vi "Logging Main.vi"() -> ()   [LabVIEW 2013]
doc: "This Continuous Measurement sample project is based on the Queued Message Handler template.\n\nThe Event Handling Loop generates messages based on user interface actions.\n\nThe Message Handling Loop processes messages generated by the Event Handling Loop, or by other messages. There are also Acquisition and Logging message handling loop subVIs, and a chart updating loop."
uses:
  Settings/Settings.ctl
  Acquisition/Hardware Configuration.ctl
  Acquisition/Signal Type.ctl
  Logging/Logging Configuration.ctl
  controls/Logging UI Data.ctl
  controls/Logging UI State.ctl
  support/Message Queue/Enqueue Message (Single).vi
  support/Message Queue/Enqueue Message (Array).vi
  <vilib>/Utility/error.llb/Error Cluster From Error Code.vi
  <vilib>/ErrorRing/Error Ring.xnode
  Acquisition/Logging Acquisition.lvlib
  Logging/Logging Logging.lvlib
  Settings/Logging Settings.lvlib
  support/User Event - Stop/Logging User Event - Stop.lvlib
  support/Message Queue/Logging Message Queue.lvlib
panel:
  out "Data":waveform(dbl)[](graph)
  in  "Settings":bool
  in  "Start":bool
  in  "Stop":bool
  out "Status":string
  in  "Exit":bool
  # "Continuous Measurement Data Logger"
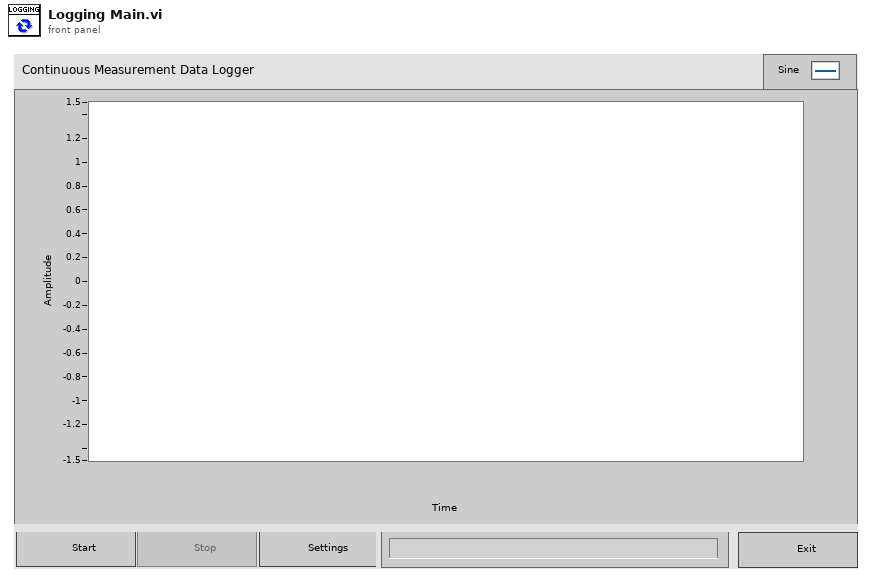
[diagram p1: front panel]
types:
  T1 = typedef "Logging UI State.ctl" = enum16{"Idle", "Acquiring and Logging", "Waiting for Exit", "Waiting for Exit (Acq Stopped)", "Waiting for Exit (Log Stopped)", "Waiting for Stop", "Waiting for Stop (Acq Stopped)", "Waiting for Stop (Log Stopped)"}
  T2 = typedef "Logging UI Data.ctl" = cluster{"Start Ref":refnum<vi>, "Stop Ref":refnum<vi>, "Settings Ref":refnum<vi>, "Exit Ref":refnum<vi>, "Status Ref":refnum<vi>, "Data Ref":refnum<vi>}
  T3 = typedef "Logging Settings.lvlib/Settings.ctl" = cluster{"Hardware Configuration":T4, "Logging Configuration":T6}
  T4 = typedef "Logging Acquisition.lvlib/Hardware Configuration.ctl" = cluster{"HW Refnum <Replace Me>":string, "Signal Type <Replace Me>":T5}
  T5 = typedef "Logging Acquisition.lvlib/Signal Type.ctl" = enum16{"Sine Wave", "Square with Noise"}
  T6 = typedef "Logging Logging.lvlib/Logging Configuration.ctl" = cluster{"Log File Base Path":path, "TDMS File Reference":refnum<k34>}
  T7 = typedef "Logging Message Queue.lvlib/All Message Queues.ctl" = cluster{"UI":refnum<queue>, "Acquisition":refnum<queue>, "Logging":refnum<queue>}
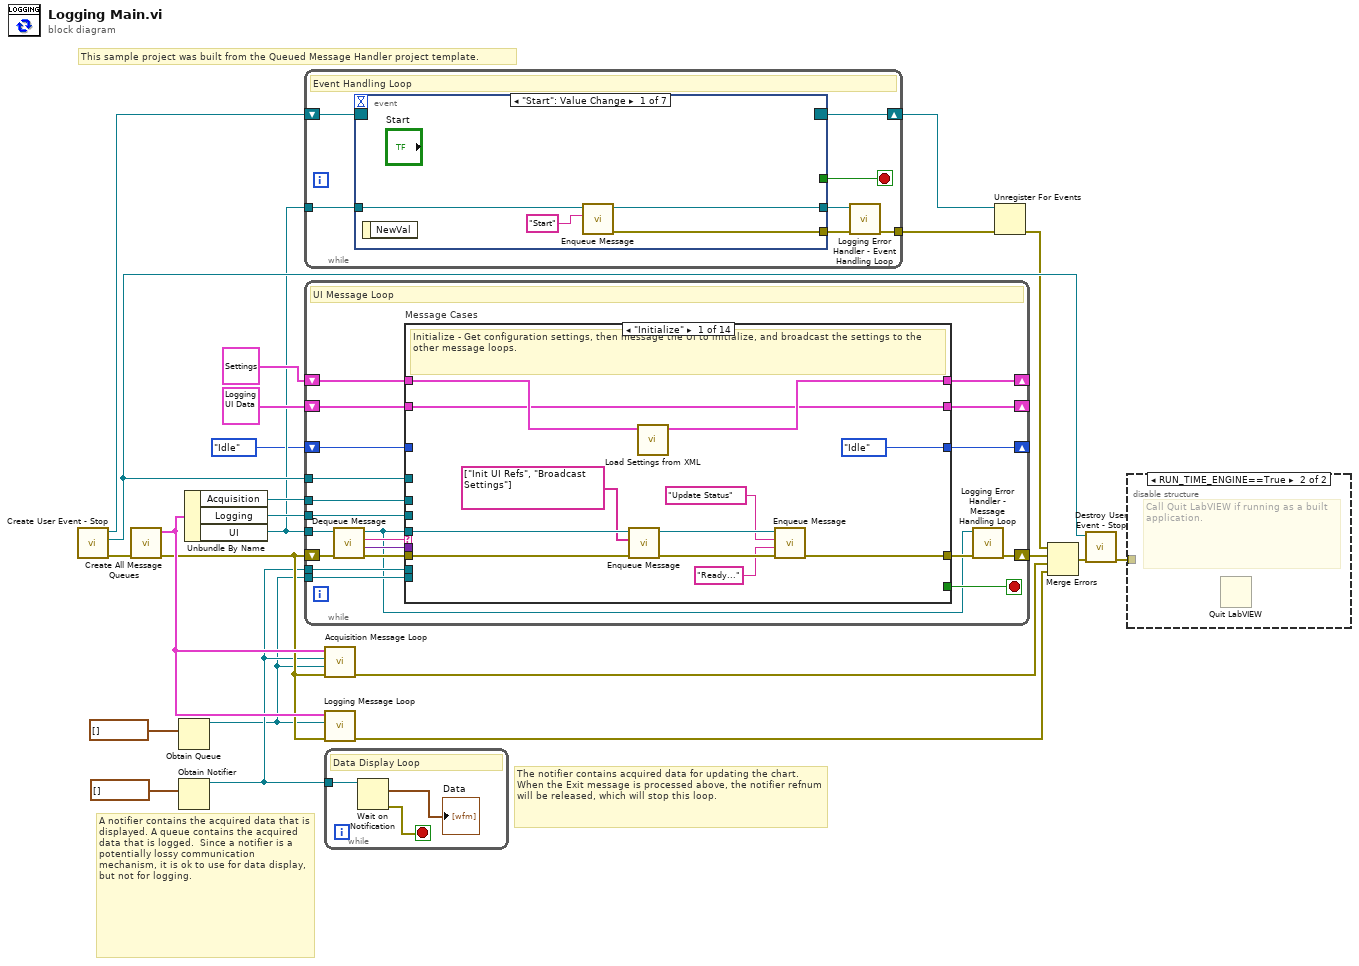
[diagram p0: block diagram]
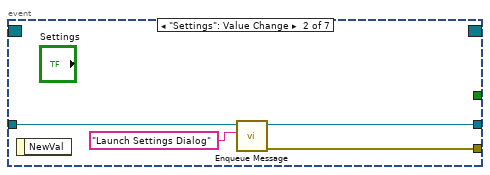
[diagram p3: hidden frame]
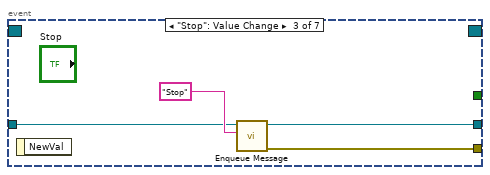
[diagram p4: hidden frame]
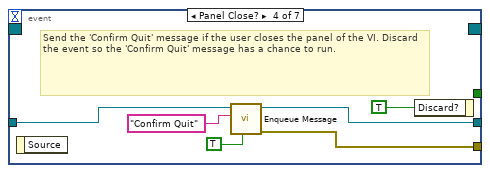
[diagram p5: hidden frame]
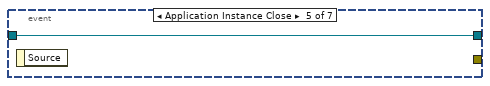
[diagram p6: hidden frame]
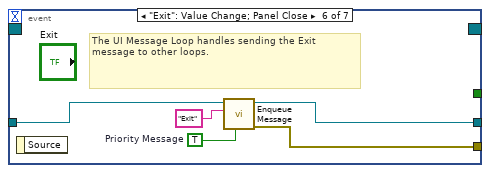
[diagram p7: hidden frame]
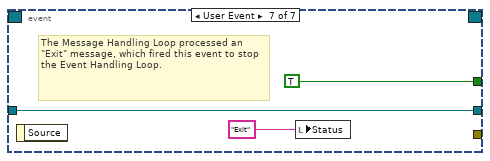
[diagram p8: hidden frame]
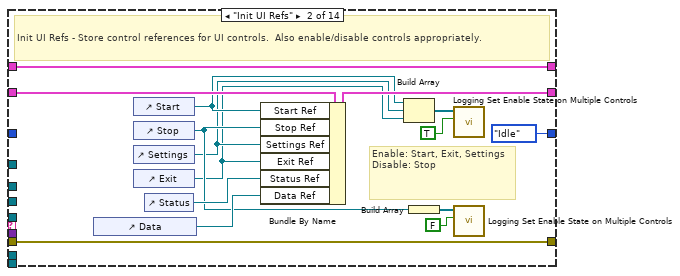
[diagram p9: hidden frame]
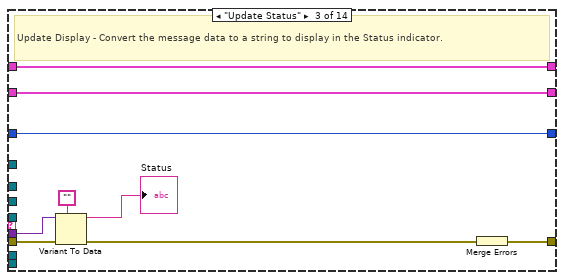
[diagram p10: hidden frame]
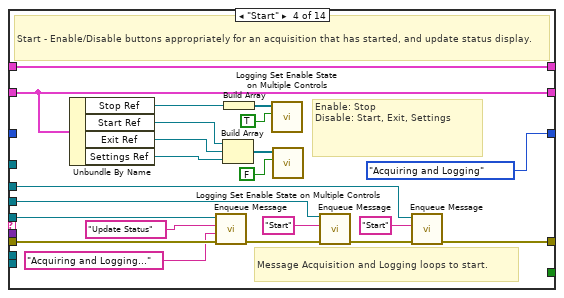
[diagram p11: hidden frame]
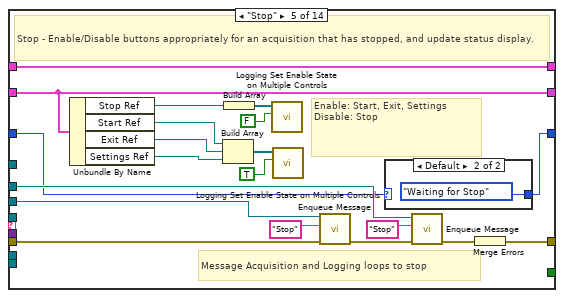
[diagram p12: hidden frame]
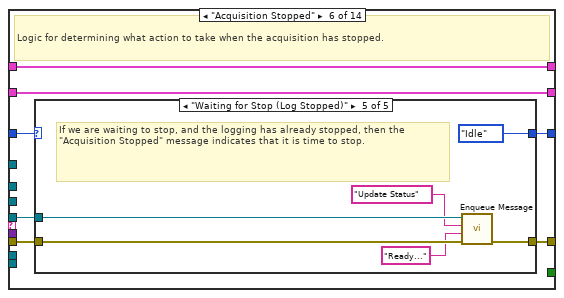
[diagram p14: hidden frame]
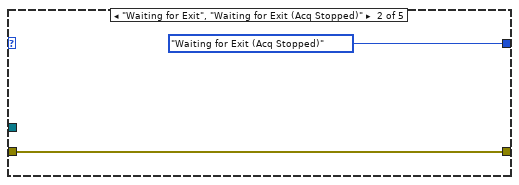
[diagram p16: hidden frame]
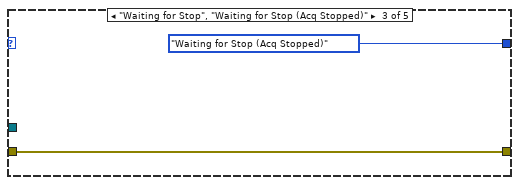
[diagram p17: hidden frame]
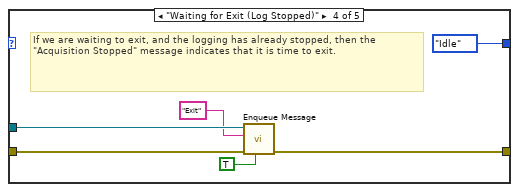
[diagram p18: hidden frame]
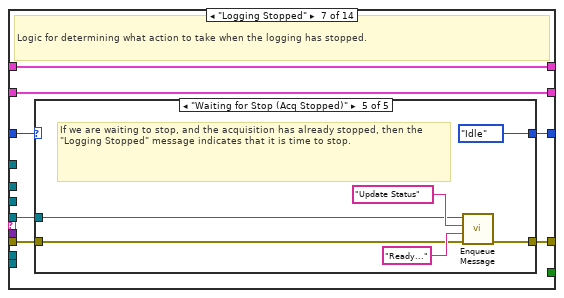
[diagram p19: hidden frame]
diagram:
  # "This sample project was built from the Queued Message Handler project template."
  # "A notifier contains the acquired data that is displayed. A queue contains the acquired data that is logged.  Since a notifier is a potentially lossy communication mechanism, it is ok to use for data display, but not for logging."
  # "The notifier contains acquired data for updating the chart. When the Exit message is processed above, the notifier refnum will be released, which will stop this loop."
  n1 = call "Create User Event - Stop.vi"() -> ("error out"=w18:errorcluster, "User Event - Stop"=w20:refnum<user-event>, "Stop Event Registration Refnum"=w21:refnum<event-registration>)  [unwired: 9 in]
  n2 = call "Create All Message Queues.vi"("error in (no error)"=w18) -> ("error out"=w15:errorcluster, "Message Queues out"=w17:T7)  [unwired: 9 in]
  n3 = Obtain Queue(element data type=waveform(dbl)[] []) -> (queue out=w4:refnum<queue>)  [unwired: 4 in, 2 out]
  n4 = Obtain Notifier(notification data type=waveform(dbl)[] []) -> (notifier out=w6:refnum<notifier>)  [unwired: 3 in, 2 out]
  n5 = Unbundle By Name(w17) -> ("Acquisition"=w10:refnum<queue>, "Logging"=w9:refnum<queue>, "UI"=w8:refnum<queue>)
  n6 = while {
    tunnel: w8 -> [w29]
    tunnel: [w26] -> w22
    shift-right: [w28] -> w12
    shift-left: w21 -> [w30]
    stop <- w27 stop-if-true
    # "Event Handling Loop"
    n7 = event shown="[0] \"Start\": Value Change" {
      selector: w30 -> [_ _ _ _ _ _ _]
      dyn-events: [_ _ _ _ _ _ _] -> w28
      timeout: _ -> [_ _ _ _ _ _ _]
      tunnel: [_ _ _ _ _ _ TRUE ("Discard?")] -> w27
      tunnel: w29 -> [w34 w36 w41 w46 w49 w51 w55]
      tunnel: [w32 w38 w40 w44 _ w54 _] -> w25
      tunnel: [w31 w35 w39 w45 w49 w50 w55] -> w24
      event "Start": Value Change {
        n8 = event-data() -> ()  [unwired: 1 in, 1 out]
        n9 = call-poly "Enqueue Message.vi"("Message"="Start", "Message Queue"=w34) -> ("error out"=w32:errorcluster, "dup Message Queue"=w31:refnum<queue>)  [unwired: 8 in]
      }
      event "Settings": Value Change {
        n10 = event-data() -> ()  [unwired: 1 in, 1 out]
        n11 = call-poly "Enqueue Message.vi"("Message"="Launch Settings Dialog", "Message Queue"=w36) -> ("error out"=w38:errorcluster, "dup Message Queue"=w35:refnum<queue>)  [unwired: 8 in]
      }
      event "Stop": Value Change {
        n12 = event-data() -> ()  [unwired: 1 in, 1 out]
        n13 = call-poly "Enqueue Message.vi"("Message"="Stop", "Message Queue"=w41) -> ("error out"=w40:errorcluster, "dup Message Queue"=w39:refnum<queue>)  [unwired: 8 in]
      }
      event Panel Close? {
        # "Send the 'Confirm Quit' message if the user closes the panel of the VI. Discard the event so the 'Confirm Quit' message has a chance to run."
        n14 = event-data() -> ()  [unwired: 1 in, 1 out]
        n15 = call-poly "Enqueue Message.vi"("Priority Message? (F)"=TRUE, "Message"="Confirm Quit", "Message Queue"=w46) -> ("error out"=w44:errorcluster, "dup Message Queue"=w45:refnum<queue>)  [unwired: 7 in]
        n16 = event-data("Discard?"=TRUE) -> ()  [unwired: 1 in, 1 out]
      }
      event Application Instance Close {
        n17 = event-data() -> ()  [unwired: 1 in, 1 out]
      }
      event "Exit": Value Change; Panel Close {
        w52 = TRUE  # Priority Message
        # "The UI Message Loop handles sending the Exit message to other loops."
        n18 = event-data() -> ()  [unwired: 1 in, 1 out]
        n19 = call-poly "Enqueue Message.vi"("Priority Message? (F)"=w52, "Message"="Exit", "Message Queue"=w51) -> ("error out"=w54:errorcluster, "dup Message Queue"=w50:refnum<queue>)  [unwired: 7 in]
      }
      event User Event {
        # "The Message Handling Loop processed an \"Exit\" message, which fired this event to stop the Event Handling Loop."
        n20 = event-data() -> ()  [unwired: 1 in, 1 out]
        n21 = local write "Status"("Exit" ("Exit String")) -> ()
      }
    }
    n22 = call "Logging Error Handler - Event Handling Loop.vi"("error in (no error)"=w25, "Message Queue"=w24) -> ("dup error in"=w26:errorcluster)  [unwired: 8 in, 1 out]
  }
  n23 = while {
    tunnel: w8 -> [w71]
    tunnel: w20 -> [w76]
    shift-right: [w62] -> w23
    shift-left: w15 -> [w75]
    shift-right: [w70] -> _
    shift-left: T3 {"Hardware Configuration"={"HW Refnum <Replace Me>"="", "Signal Type <Replace Me>"=enum."Sine Wave"}, "Logging Configuration"={"Log File Base Path"=path "", "TDMS File Reference"=refnum}} ("Settings") -> [w69]
    shift-right: [w67] -> _
    shift-left: T2 {"Start Ref"=refnum, "Stop Ref"=refnum, "Settings Ref"=refnum, "Exit Ref"=refnum, "Status Ref"=refnum, "Data Ref"=refnum} ("Measurement UI Controls") -> [w68]
    tunnel: w10 -> [w66]
    tunnel: w9 -> [w65]
    tunnel: w6 -> [w64]
    tunnel: w4 -> [w63]
    shift-right: [w58] -> _
    shift-left: Logging_UI_State."Idle" ("UI State") -> [w59]
    stop <- w77 stop-if-true
    # "UI Message Loop"
    n24 = call "Dequeue Message.vi"("error in (no error)"=w75, "Message Queue"=w71) -> ("error out"=w74:errorcluster, "Message Data"=w72:variant, "Message"=w73:string, "dup Message Queue"=w60:refnum<queue>)  [unwired: 6 in]
    n25 = case "Message Cases" shown="\"Initialize\"" w73 {
      selector: w73 -> [_ _ _ _ _ _ _ _ _ _ _ _ _ w298]
      tunnel: w60 -> [w81 _ _ w135 _ w160 w185 _ w225 w239 w250 w281 _ _]
      tunnel: w74 -> [w80 w104 w112 w134 w154 w161 w186 w213 w227 w242 w249 w289 w296 _]
      tunnel: [w85 w104 w113 w117 w155 w158 w183 w219 w222 w238 w248 w290 w295 w297] -> w61
      tunnel: [_ _ _ _ _ _ _ _ _ _ _ TRUE _ _] -> w77
      tunnel: w72 -> [_ _ w111 _ _ _ _ _ _ w240 _ _ _ _]
      tunnel: w76 -> [_ _ _ _ _ _ _ _ _ _ _ w288 _ _]
      tunnel: [w88 w103 w107 w133 w153 w164 w189 w217 w224 w246 w253 w286 w294 w301] -> w70
      tunnel: w69 -> [w89 w103 w107 w133 w153 w164 w189 w217 w228 w246 w253 w286 w294 w301]
      tunnel: w68 -> [w82 w102 w106 w130 w152 w163 w188 w211 w221 w245 w252 w284 w293 w300]
      tunnel: [w82 w99 w106 w130 w152 w163 w188 w211 w221 w245 w252 w284 w293 w300] -> w67
      tunnel: w66 -> [_ _ _ w116 w139 _ _ w210 _ _ _ w283 _ _]
      tunnel: w65 -> [_ _ _ w119 w142 _ _ w209 _ _ _ w282 _ _]
      tunnel: w64 -> [_ _ _ _ _ _ _ _ _ _ _ w280 _ _]
      tunnel: w63 -> [_ _ _ _ _ _ _ _ _ _ _ w276 _ _]
      tunnel: w59 -> [_ _ w105 _ w136 w162 w187 w208 w220 w234 w251 _ w292 w299]
      tunnel: [Logging_UI_State."Idle" ("UI State") Logging_UI_State."Idle" ("UI State") w105 Logging_UI_State."Acquiring and Logging" ("UI State") w137 w159 w184 w208 w220 w234 w247 Logging_UI_State."Idle" ("UI State") w292 w299] -> w58
      frame "Initialize" {
        # "Initialize - Get configuration settings, then message the UI to initialize, and broadcast the settings to the other message loops."
        n26 = call-poly "Enqueue Message.vi"("error in (no error)"=w80, "Message Array"=string[] ["Init UI Refs", "Broadcast Settings"], "Message Queue"=w81) -> ("error out"=w87:errorcluster, "dup Message Queue"=w86:refnum<queue>)  [unwired: 7 in]
        n27 = call "Load Settings from XML.vi"("Settings in"=w89) -> ("Settings out"=w88:T3)  [unwired: 9 in, 1 out]
        n28 = call-poly "Enqueue Message.vi"("error in (no error)"=w87, "Message Data"="Ready..." ("Ready..."), "Message"="Update Status", "Message Queue"=w86) -> ("error out"=w85:errorcluster)  [unwired: 6 in, 1 out]
      }
      frame "Init UI Refs" {
        # "Enable: Start, Exit, Settings\nDisable: Stop"
        # "Init UI Refs - Store control references for UI controls.  Also enable/disable controls appropriately."
        n29 = control-ref of="Data"() -> (w100:refnum<vi>)
        n30 = control-ref of="Start"() -> (w93:refnum<vi>)
        n31 = control-ref of="Stop"() -> (w94:refnum<vi>)
        n32 = control-ref of="Settings"() -> (w92:refnum<vi>)
        n33 = control-ref of="Exit"() -> (w91:refnum<vi>)
        n34 = control-ref of="Status"() -> (w101:refnum<vi>)
        n35 = Bundle By Name(cluster=w102, "Start Ref"=w93, "Stop Ref"=w94, "Settings Ref"=w92, "Exit Ref"=w91, "Status Ref"=w101, "Data Ref"=w100) -> (w99:T2)
        n36 = Build Array(w93, w92, w91) -> (w97:refnum<vi>[])
        n37 = Build Array(w94) -> (w96:refnum<vi>[])
        n38 = call "Logging Set Enable State on Multiple Controls.vi"("Enable?"=TRUE, "Controls"=w97) -> ()  [unwired: 10 in]
        n39 = call "Logging Set Enable State on Multiple Controls.vi"("Enable?"=FALSE, "Controls"=w96) -> ()  [unwired: 10 in]
      }
      frame "Update Status" {
        # "Update Display - Convert the message data to a string to display in the Status indicator."
        n40 = Variant To Data(error in=w112, type="", Variant=w111) -> (data=→"Status":string, error out=w109:errorcluster)
        n41 = Merge Errors(w109) -> (w113:errorcluster)
      }
      frame "Start" {
        # "Message Acquisition and Logging loops to start."
        # "Enable: Stop\nDisable: Start, Exit, Settings"
        # "Start - Enable/Disable buttons appropriately for an acquisition that has started, and update status display."
        n42 = Unbundle By Name(w130) -> ("Stop Ref"=w125:refnum<vi>, "Start Ref"=w124:refnum<vi>, "Exit Ref"=w123:refnum<vi>, "Settings Ref"=w122:refnum<vi>)
        n43 = call-poly "Enqueue Message.vi"("error in (no error)"=w134, "Message Data"="Acquiring and Logging..." ("Acquiring and Logging..."), "Message"="Update Status", "Message Queue"=w135) -> ("error out"=w121:errorcluster)  [unwired: 6 in, 1 out]
        n44 = Build Array(w124, w123, w122) -> (w128:refnum<vi>[])
        n45 = Build Array(w125) -> (w127:refnum<vi>[])
        n46 = call "Logging Set Enable State on Multiple Controls.vi"("Enable?"=TRUE, "Controls"=w127) -> ()  [unwired: 10 in]
        n47 = call "Logging Set Enable State on Multiple Controls.vi"("Enable?"=FALSE, "Controls"=w128) -> ()  [unwired: 10 in]
        n48 = call-poly "Enqueue Message.vi"("error in (no error)"=w121, "Message"="Start", "Message Queue"=w119) -> ("error out"=w118:errorcluster)  [unwired: 7 in, 1 out]
        n49 = call-poly "Enqueue Message.vi"("error in (no error)"=w118, "Message"="Start", "Message Queue"=w116) -> ("error out"=w117:errorcluster)  [unwired: 7 in, 1 out]
      }
      frame "Stop" {
        # "Message Acquisition and Logging loops to stop"
        # "Enable: Start, Exit, Settings\nDisable: Stop"
        # "Stop - Enable/Disable buttons appropriately for an acquisition that has stopped, and update status display."
        n50 = Unbundle By Name(w152) -> ("Stop Ref"=w147:refnum<vi>, "Start Ref"=w146:refnum<vi>, "Exit Ref"=w145:refnum<vi>, "Settings Ref"=w144:refnum<vi>)
        n51 = Build Array(w146, w145, w144) -> (w150:refnum<vi>[])
        n52 = Build Array(w147) -> (w149:refnum<vi>[])
        n53 = call "Logging Set Enable State on Multiple Controls.vi"("Enable?"=FALSE, "Controls"=w149) -> ()  [unwired: 10 in]
        n54 = call "Logging Set Enable State on Multiple Controls.vi"("Enable?"=TRUE, "Controls"=w150) -> ()  [unwired: 10 in]
        n55 = call-poly "Enqueue Message.vi"("error in (no error)"=w154, "Message"="Stop", "Message Queue"=w142) -> ("error out"=w141:errorcluster)  [unwired: 7 in, 1 out]
        n56 = case shown="Default" w136 {
          selector: w136 -> [w156 _]
          tunnel: [w156 Logging_UI_State."Waiting for Stop" ("UI State")] -> w137
          frame "Waiting for Exit" {
          }
          frame Default {
          }
        }
        n57 = call-poly "Enqueue Message.vi"("error in (no error)"=w141, "Message"="Stop", "Message Queue"=w139) -> ("error out"=w140:errorcluster)  [unwired: 7 in, 1 out]
        n58 = Merge Errors(w140) -> (w155:errorcluster)
      }
      frame "Acquisition Stopped" {
        # "Logic for determining what action to take when the acquisition has stopped."
        n59 = case shown="\"Waiting for Stop (Log Stopped)\"" w162 {
          selector: w162 -> [w166 _ _ _ _]
          tunnel: w161 -> [w165 w168 w170 w176 w182]
          tunnel: w160 -> [_ _ _ w174 w179]
          tunnel: [w166 Logging_UI_State."Waiting for Exit (Acq Stopped)" ("UI State") Logging_UI_State."Waiting for Stop (Acq Stopped)" ("UI State") Logging_UI_State."Idle" ("UI State") Logging_UI_State."Idle" ("UI State")] -> w159
          tunnel: [w165 w168 w170 w175 w180] -> w158
          frame Default {
          }
          frame "Waiting for Exit", "Waiting for Exit (Acq Stopped)" {
          }
          frame "Waiting for Stop", "Waiting for Stop (Acq Stopped)" {
          }
          frame "Waiting for Exit (Log Stopped)" {
            # "If we are waiting to exit, and the logging has already stopped, then the \"Acquisition Stopped\" message indicates that it is time to exit."
            n60 = call-poly "Enqueue Message.vi"("Priority Message? (F)"=TRUE, "error in (no error)"=w176, "Message"="Exit", "Message Queue"=w174) -> ("error out"=w175:errorcluster)  [unwired: 6 in, 1 out]
          }
          frame "Waiting for Stop (Log Stopped)" {
            # "If we are waiting to stop, and the logging has already stopped, then the \"Acquisition Stopped\" message indicates that it is time to stop."
            n61 = call-poly "Enqueue Message.vi"("error in (no error)"=w182, "Message Data"="Ready..." ("Ready..."), "Message"="Update Status", "Message Queue"=w179) -> ("error out"=w180:errorcluster)  [unwired: 6 in, 1 out]
          }
        }
      }
      frame "Logging Stopped" {
        # "Logic for determining what action to take when the logging has stopped."
        n62 = case shown="\"Waiting for Stop (Acq Stopped)\"" w187 {
          selector: w187 -> [w191 _ _ _ _]
          tunnel: w186 -> [w190 w193 w195 w201 w204]
          tunnel: w185 -> [_ _ _ w199 w203]
          tunnel: [w191 Logging_UI_State."Waiting for Exit (Log Stopped)" ("UI State") Logging_UI_State."Waiting for Stop (Log Stopped)" ("UI State") Logging_UI_State."Idle" ("UI State") Logging_UI_State."Idle" ("UI State")] -> w184
          tunnel: [w190 w193 w195 w200 w202] -> w183
          frame Default {
          }
          frame "Waiting for Exit", "Waiting for Exit (Log Stopped)" {
          }
          frame "Waiting for Stop", "Waiting for Stop (Log Stopped)" {
          }
          frame "Waiting for Exit (Acq Stopped)" {
            # "If we are waiting to exit, and the acquisition has already stopped, then the \"Logging Stopped\" message indicates that it is time to exit."
            n63 = call-poly "Enqueue Message.vi"("Priority Message? (F)"=TRUE, "error in (no error)"=w201, "Message"="Exit", "Message Queue"=w199) -> ("error out"=w200:errorcluster)  [unwired: 6 in, 1 out]
          }
          frame "Waiting for Stop (Acq Stopped)" {
            # "If we are waiting to stop, and the acquisition has already stopped, then the \"Logging Stopped\" message indicates that it is time to stop."
            n64 = call-poly "Enqueue Message.vi"("error in (no error)"=w204, "Message Data"="Ready..." ("Ready..."), "Message"="Update Status", "Message Queue"=w203) -> ("error out"=w202:errorcluster)  [unwired: 6 in, 1 out]
          }
        }
      }
      frame "Broadcast settings" {
        w212 = "Update Settings" ("Message")
        # "Broadcast settings - Send the 'Update Settings' message to the Logging and Acquisition message loops."
        n65 = Unbundle By Name(w217) -> ("Hardware Configuration"=w216:T4, "Logging Configuration"=w215:T6)
        n66 = call-poly "Enqueue Message.vi"("Message Data"=w216, "Message"=w212, "Message Queue"=w210) -> ("error out"=w218:errorcluster)  [unwired: 7 in, 1 out]
        n67 = call-poly "Enqueue Message.vi"("error in (no error)"=w218, "Message Data"=w215, "Message"=w212, "Message Queue"=w209) -> ("error out"=w214:errorcluster)  [unwired: 6 in, 1 out]
        n68 = Merge Errors(w214, w213) -> (w219:errorcluster)
      }
      frame "Launch Settings Dialog" {
        # "Launch Settings Dialog - Launch the Settings Dialog when the user clicks the 'Settings' button."
        n69 = call "Settings Dialog.vi"("error in (no error)"=w227, "Settings in"=w228) -> ("error out"=w223:errorcluster, "Cancelled?"=w226:bool, "Settings out"=w224:T3)  [unwired: 6 in, 1 out]
        n70 = case shown="False" w226 {
          tunnel: w225 -> [w232 _]
          tunnel: w223 -> [w231 w233]
          tunnel: [w230 w233] -> w222
          frame False {
            n71 = call-poly "Enqueue Message.vi"("error in (no error)"=w231, "Message"="Broadcast Settings", "Message Queue"=w232) -> ("error out"=w230:errorcluster)  [unwired: 7 in, 1 out]
          }
          frame True {
          }
        }
      }
      frame "Error" {
        # "Error - Check the error message data and respond accordingly. This message is sent by the \"Error Handler\" VIs at the end of each loop in this application."
        n72 = Variant To Data(error in=w242, type=errorcluster {"status"=FALSE, "code"=0, "source"=""} ("error constant"), Variant=w240) -> (data=w244:errorcluster, error out=w241:errorcluster)
        n73 = call <vilib>:"Simple Error Handler.vi"("error in (no error)"=w244) -> ()  [unwired: 4 in, 5 out]
        n74 = call-poly "Enqueue Message.vi"("Priority Message? (F)"=TRUE, "Message"="Exit", "Message Queue"=w239) -> ("error out"=w237:errorcluster)  [unwired: 7 in, 1 out]
        n75 = Merge Errors(w237, w241) -> (w238:errorcluster)
      }
      frame "Confirm Quit" {
        # "Confirm Quit - Message that can confirm whether or not the user wants to exit the application."
        n76 = case shown="\"Acquiring and Logging\"" w251 {
          tunnel: w250 -> [w259 w263]
          tunnel: w249 -> [w258 w262]
          tunnel: [w257 w261] -> w248
          tunnel: [Logging_UI_State."Idle" ("UI State") w260] -> w247
          frame Default {
            # "If 'Confirm Quit' comes in while the system is idle, there is no need for a confirmation message."
            n77 = call-poly "Enqueue Message.vi"("Priority Message? (F)"=TRUE, "error in (no error)"=w258, "Message"="Exit", "Message Queue"=w259) -> ("error out"=w257:errorcluster)  [unwired: 6 in, 1 out]
          }
          frame "Acquiring and Logging" {
            n78 = Two Button Dialog(message="Are you sure you want to quit while the acquisition is running?" ("Confirm Quit Message"), 1:"No" ("No"), 2:"Yes" ("Yes")) -> (T button?=w264:bool)
            n79 = case shown="True" w264 {
              tunnel: w263 -> [_ w273]
              tunnel: w262 -> [w269 w274]
              tunnel: [w269 w272] -> w261
              tunnel: [Logging_UI_State."Acquiring and Logging" ("UI State") Logging_UI_State."Waiting for Exit" ("UI State")] -> w260
              frame False {
                # "User did not want to quit."
              }
              frame True {
                n80 = call-poly "Enqueue Message.vi"("error in (no error)"=w274, "Message"="Stop", "Message Queue"=w273) -> ("error out"=w272:errorcluster)  [unwired: 7 in, 1 out]
              }
            }
          }
        }
      }
      frame "Exit" {
        w285 = "Exit" ("Message")
        # "Don't check the error outs. The acquisition and logging queues may have already been released."
        # "Close references owned by the Main VI."
        # "Stop the VI"
        # "Exit - Fire the User Event to stop the Event Handling Loop.  Also send Exit messages to the Acquisition and Logging loops."
        n81 = Release Queue(queue=w281, error in (no error)=w289) -> (error out=w279:errorcluster)  [unwired: 1 in, 2 out]
        n82 = call "Fire User Event - Stop.vi"("User Event - Stop"=w288) -> ("error out"=w287:errorcluster)  [unwired: 10 in]
        n83 = Release Notifier(notifier=w280, error in (no error)=w279) -> (error out=w278:errorcluster)  [unwired: 1 in, 2 out]
        n84 = Release Queue(queue=w276, error in (no error)=w278) -> (error out=w277:errorcluster)  [unwired: 1 in, 2 out]
        n85 = call-poly "Enqueue Message.vi"("Message"=w285, "Message Queue"=w283) -> ()  [unwired: 8 in, 2 out]
        n86 = call-poly "Enqueue Message.vi"("Message"=w285, "Message Queue"=w282) -> ()  [unwired: 8 in, 2 out]
        n87 = Merge Errors(w287, w277) -> (w290:errorcluster)
      }
      frame "---Copy This Frame---" {
        # "Duplicate this frame when creating new messages.  Change this comment in the duplicated frame to describe this message."
        n88 = Merge Errors(w296) -> (w295:errorcluster)
      }
      frame Default {
        # "'Default' case only runs if there is a message that isn't defined in any of the other cases.  Output a programming error."
        n89 = xnode "Error Ring"("parameter 0"=w298) -> ("error out"=w297:errorcluster)
      }
    }
    n90 = call "Logging Error Handler - Message Handling Loop.vi"("error in (no error)"=w61, "Message Queue"=w60) -> ("dup error in"=w62:errorcluster)  [unwired: 8 in, 1 out]
  }
  n91 = call "Acquisition Message Loop.vi"("error in (no error)"=w15, "Data Queue"=w4, "Data Notifier"=w6, "Message Queues"=w17) -> ("error out"=w19:errorcluster)  [unwired: 7 in]
  n92 = call "Logging Message Loop.vi"("error in (no error)"=w15, "Data Queue"=w4, "Message Queues"=w17) -> ("error out"=w16:errorcluster)  [unwired: 8 in]
  n93 = while "Data Display Loop" {
    tunnel: w6 -> [w311]
    stop <- w309 stop-if-true
    # "Data Display Loop"
    n94 = Wait on Notification(notifier=w311) -> (notification=→"Data":waveform(dbl)[], error out=w309:errorcluster)  [unwired: 3 in, 2 out]
  }
  n95 = Unregister For Events(event registration refnum=w12, error in=w22) -> (error out=w13:errorcluster)
  n96 = Merge Errors(w13, w23, w19, w16) -> (w1:errorcluster)
  n97 = call "Destroy User Event - Stop.vi"("error in (no error)"=w1, "User Event - Stop"=w20) -> ("error out"=w3:errorcluster)  [unwired: 9 in]
  n98 = disable-structure shown="RUN_TIME_ENGINE==True" {
    disable-tunnel: w3 -> [_ _]
    frame condition #0 (active) {
    }
    frame condition #1 {
      # "Call Quit LabVIEW if running as a built application."
      n99 = Quit LabVIEW() -> ()  [unwired: 1 in]
    }
  }
